vi "Format.vi"(6 "Statement":T1={"timestamp"=timestamp(0 s since 1904-01-01), "level"=enum."INFO", "sourceTag"="", "originVI"="", "message"=""}, 8 "error in (no error)":errorcluster, 11 "JSONLayout in":refnum<class "JSONLayout.lvclass">) -> (0 "error out":errorcluster, 3 "JSONLayout out":refnum<class "JSONLayout.lvclass">, 4 "FormattedLine":string)   [LabVIEW 2026, in "Lumberjack.lvlib" / "JSONLayout.lvclass"]
doc: "Overrides Layout.Format. Emits one JSON object per statement in the Go slog convention: time (ISO 8601 via FormatTimeString, framed by useUTC), level (UPPERCASE Severity token), msg, then the sourceTag and originVI attributes, omitted when empty. Values are escaped by JSONEscapeString; keys are fixed literals. Content only, no trailing terminator, so a file of these lines is JSON Lines."
uses:
  JSONLayout.lvclass
  C:/Users/dallis/OneDrive - Velico Medical/Documents/Personal/LabVIEW Coding Projects/Lumberjack/src/Core/Layouts/Layout.lvclass/Layout.lvclass
  TypeDefs/Statement.ctl
  TypeDefs/Severity.ctl
  Layout.lvclass/Layout.lvclass
  Lumberjack.lvlib
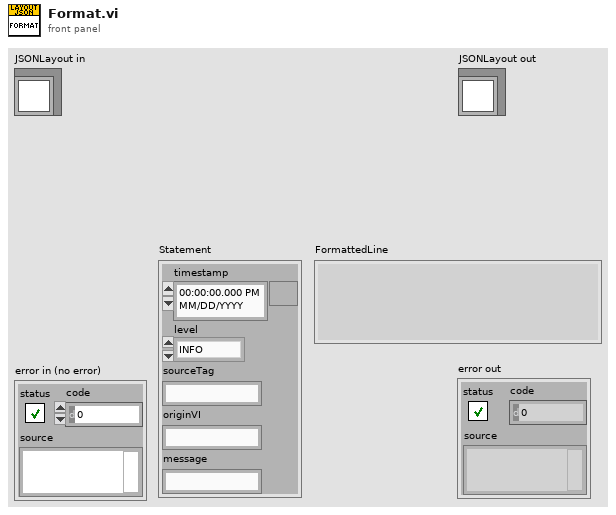
[diagram p1: front panel]
types:
  T1 = typedef "Lumberjack.lvlib/Statement.ctl" = cluster{"timestamp":timestamp, "level":T2, "sourceTag":string, "originVI":string, "message":string}
  T2 = typedef "Lumberjack.lvlib/Severity.ctl" = enum16{"OFF", "FATAL", "ERROR", "WARN", "INFO", "DEBUG", "TRACE", "ALL"}
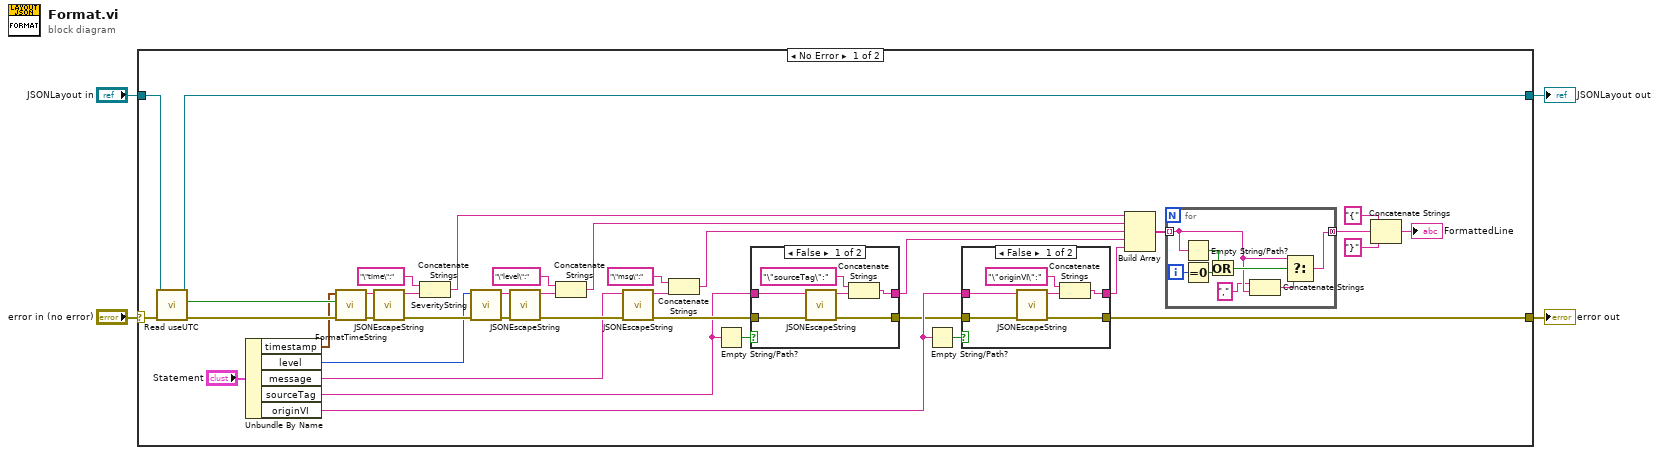
[diagram p0: block diagram]
diagram:
  n1 = case shown="No Error" "error in (no error)" {
    selector: "error in (no error)" -> [w41 w68]
    tunnel: "JSONLayout in" -> [w42 w67]
    tunnel: [w9 w68] -> w2
    tunnel: [w11 w67] -> w1
    frame No Error {
      n2 = call "Read useUTC.vi"("error in (no error)"=w41, "Layout in"=w42) -> ("error out"=w40:errorcluster, "useUTC"=w39:bool, "Layout out"=w11:refnum<class "JSONLayout.lvclass">)  [unwired: 7 in]
      n3 = Unbundle By Name("Statement") -> ("timestamp"=w27:timestamp, "level"=w24:T2, "message"=w23:string, "sourceTag"=w21:string, "originVI"=w19:string)
      n4 = call "FormatTimeString.vi"("error in (no error)"=w40, "useUTC"=w39, "timestamp"=w27) -> ("error out"=w36:errorcluster, "timeString"=w35:string)  [unwired: 7 in]
      n5 = call "JSONEscapeString.vi"("error in (no error)"=w36, "raw"=w35) -> ("error out"=w32:errorcluster, "escaped"=w34:string)  [unwired: 8 in]
      n6 = Concatenate Strings("\"time\":", w34) -> (w16:string)
      n7 = call "SeverityString.vi"("error in (no error)"=w32, "Severity"=w24) -> ("error out"=w33:errorcluster, "SeverityString"=w31:string)  [unwired: 8 in]
      n8 = call "JSONEscapeString.vi"("error in (no error)"=w33, "raw"=w31) -> ("error out"=w28:errorcluster, "escaped"=w30:string)  [unwired: 8 in]
      n9 = Concatenate Strings("\"level\":", w30) -> (w15:string)
      n10 = call "JSONEscapeString.vi"("error in (no error)"=w28, "raw"=w23) -> ("error out"=w22:errorcluster, "escaped"=w26:string)  [unwired: 8 in]
      n11 = Concatenate Strings("\"msg\":", w26) -> (w14:string)
      n12 = Empty String/Path?(string/path=w21) -> (empty?=w20:bool)
      n13 = case shown="False" w20 {
        tunnel: w22 -> [w64 w65]
        tunnel: [w63 w65] -> w17
        tunnel: w21 -> [w60 w66]
        tunnel: [w59 w66] -> w13
        frame False {
          n14 = call "JSONEscapeString.vi"("error in (no error)"=w64, "raw"=w60) -> ("error out"=w63:errorcluster, "escaped"=w62:string)  [unwired: 8 in]
          n15 = Concatenate Strings("\"sourceTag\":", w62) -> (w59:string)
        }
        frame True {
        }
      }
      n16 = Empty String/Path?(string/path=w19) -> (empty?=w18:bool)
      n17 = case shown="False" w18 {
        tunnel: w17 -> [w56 w57]
        tunnel: [w55 w57] -> w9
        tunnel: w19 -> [w52 w58]
        tunnel: [w51 w58] -> w12
        frame False {
          n18 = call "JSONEscapeString.vi"("error in (no error)"=w56, "raw"=w52) -> ("error out"=w55:errorcluster, "escaped"=w54:string)  [unwired: 8 in]
          n19 = Concatenate Strings("\"originVI\":", w54) -> (w51:string)
        }
        frame True {
        }
      }
      n20 = Build Array(w16, w15, w14, w13, w12) -> (w10:string[])
      n21 = for {
        tunnel: w10 -> [w44] mode=indexing
        tunnel: [w45] -> w8 mode=concatenating
        i -> [w50]
        n22 = Empty String/Path?(string/path=w44) -> (empty?=w46:bool)
        n23 = Equal To 0?(x=w50) -> (x = 0?=w49:bool)
        n24 = Or(x=w46, y=w49) -> (x .or. y?=w47:bool)
        n25 = Concatenate Strings("," ("string"), w44) -> (w48:string)
        n26 = Select(t=w44, s=w47, f=w48) -> (s? t:f=w45:string)
      }
      n27 = Concatenate Strings("{" ("string"), w8, "}" ("string")) -> (→"FormattedLine":string)
    }
    frame Error {
    }
  }
  "error out" <- w2
  "JSONLayout out" <- w1
